vi "3-4.vi"(2 "字符串 3":string, 3 "数值":dbl, 4 "字符串":string) -> (0 "长度":i32, 1 "结果字符串":string)   [LabVIEW 2017]
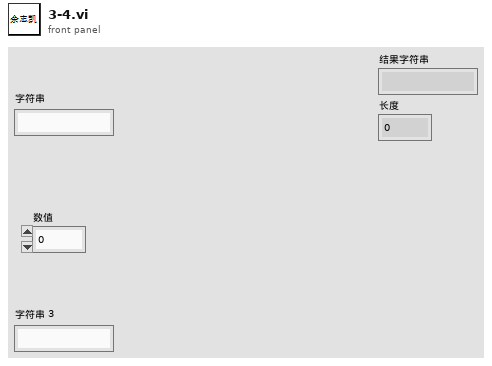
[diagram p1: front panel]
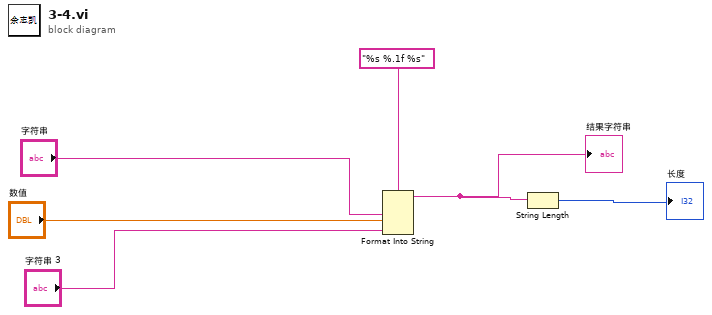
[diagram p0: block diagram]
diagram:
  n1 = Format Into String(format string="%s %.1f %s" ("格式字符串"), "字符串", "数值", "字符串 3") -> (resulting string=w4:string)  [unwired: 2 in, 1 out]
  "结果字符串" <- w4
  n2 = String Length(string=w4) -> (length=→"长度":i32)
